vi "GeoData.vi"() -> ()   [LabVIEW 2017] (continued)
H1\n47264\t18105\tNorman\tIN\tMonroe County\tH1\n47460\t18105\tSpencer\tIN\tMonroe County\tH1\n47426\t18105\tClear creek\tIN\tMonroe County\tH1\n47434\t18105\tHarrodsburg\tIN\tMonroe County\tH1\n47463\t18105\tStanford\tIN\tMonroe County\tH1\n47458\t18105\tSmithville\tIN\tMonroe County\tH1\n47402\t18105\tBloomington\tIN\tMonroe County\tH1\n46151\t18105\tMartinsville\tIN\tMonroe County\tH1\n47990\t18107\tWaynetown\tIN\tMontgomery County\tH1\n46035\t18107\tColfax\tIN\tMontgomery County\tH1\n47954\t18107\tLadoga\tIN\tMontgomery County\tH1\n46175\t18107\tRussellville\tIN\tMontgomery County\tH1\n47955\t18107\tLinden\tIN\tMontgomery County\tH1\n47933\t18107\tCrawfordsville\tIN\tMontgomery County\tH1\n47968\t18107\tNew ross\tIN\tMontgomery County\tH1\n47967\t18107\tNew richmond\tIN\tMontgomery County\tH1\n47994\t18107\tWingate\tIN\tMontgomery County\tH1\n47949\t18107\tHillsboro\tIN\tMontgomery County\tH1\n47916\t18107\tAlamo\tIN\tMontgomery County\tH1\n47981\t18107\tRomney\tIN\tMontgomery County\tH1\n47940\t18107\tDarlington\tIN\tMontgomery County\tH1\n47989\t18107\tWaveland\tIN\tMontgomery County\tH1\n46071\t18107\tThorntown\tIN\tMontgomery County\tH1\n47930\t18107\tClarks hill\tIN\tMontgomery County\tH1\n47965\t18107\tNew market\tIN\tMontgomery County\tH1\n46158\t18109\tMooresville\tIN\tMorgan County\tH1\n46166\t18109\tParagon\tIN\tMorgan County\tH1\n46106\t18109\tBargersville\tIN\tMorgan County\tH1\n47433\t18109\tGosport\tIN\tMorgan County\tH1\n46120\t18109\tCloverdale\tIN\tMorgan County\tH1\n46111\t18109\tBrooklyn\tIN\tMorgan County\tH1\n46157\t18109\tMonrovia\tIN\tMorgan County\tH1\n46113\t18109\tCamby\tIN\tMorgan County\tH1\n46125\t18109\tEminence\tIN\tMorgan County\tH1\n46180\t18109\tStilesville\tIN\tMorgan County\tH1\n46160\t18109\tMorgantown\tIN\tMorgan County\tH1\n46118\t18109\tClayton\tIN\tMorgan County\tH1\n46151\t18109\tMartinsville\tIN\tMorgan County\tH1\n47456\t18109\tQuincy\tIN\tMorgan County\tH1\n46310\t18111\tDemotte\tIN\tNewton County\tH1\n46379\t18111\tSumava resorts\tIN\tNewton County\tH1\n46372\t18111\tRoselawn\tIN\tNewton County\tH1\n46349\t18111\tLake village\tIN\tNewton County\tH1\n47978\t18111\tRensselaer\tIN\tNewton County\tH1\n46341\t18111\tHebron\tIN\tNewton County\tH1\n47948\t18111\tGoodland\tIN\tNewton County\tH1\n47942\t18111\tEarl park\tIN\tNewton County\tH1\n47922\t18111\tBrook\tIN\tNewton County\tH1\n47963\t18111\tMorocco\tIN\tNewton County\tH1\n47964\t18111\tMount ayr\tIN\tNewton County\tH1\n46381\t18111\tThayer\tIN\tNewton County\tH1\n47951\t18111\tKentland\tIN\tNewton County\tH1\n47943\t18111\tFair oaks\tIN\tNewton County\tH1\n46725\t18113\tColumbia city\tIN\tNoble County\tH1\n46760\t18113\tKimmell\tIN\tNoble County\tH1\n46732\t18113\tCromwell\tIN\tNoble County\tH1\n46796\t18113\tWolflake\tIN\tNoble County\tH1\n46730\t18113\tCorunna\tIN\tNoble County\tH1\n46748\t18113\tHuntertown\tIN\tNoble County\tH1\n46794\t18113\tWawaka\tIN\tNoble County\tH1\n46562\t18113\tPierceton\tIN\tNoble County\tH1\n46755\t18113\tKendallville\tIN\tNoble County\tH1\n46571\t18113\tTopeka\tIN\tNoble County\tH1\n46764\t18113\tLarwill\tIN\tNoble County\tH1\n46701\t18113\tAlbion\tIN\tNoble County\tH1\n46710\t18113\tAvilla\tIN\tNoble County\tH1\n46784\t18113\tRome city\tIN\tNoble County\tH1\n46543\t18113\tMillersburg\tIN\tNoble County\tH1\n46763\t18113\tLaotto\tIN\tNoble County\tH1\n46767\t18113\tLigonier\tIN\tNoble County\tH1\n46723\t18113\tChurubusco\tIN\tNoble County\tH1\n46795\t18113\tWolcottville\tIN\tNoble County\tH1\n47001\t18115\tAurora\tIN\tOhio County\tH1\n47018\t18115\tDillsboro\tIN\tOhio County\tH1\n47038\t18115\tPatriot\tIN\tOhio County\tH1\n47011\t18115\tBennington\tIN\tOhio County\tH1\n47040\t18115\tRising sun\tIN\tOhio County\tH1\n47017\t18115\tCross plains\tIN\tOhio County\tH1\n47108\t18117\tCampbellsburg\tIN\tOrange County\tH1\n47175\t18117\tTaswell\tIN\tOrange County\tH1\n47469\t18117\tWest baden springs\tIN\tOrange County\tH1\n47452\t18117\tOrleans\tIN\tOrange County\tH1\n47446\t18117\tMitchell\tIN\tOrange County\tH1\n47454\t18117\tPaoli\tIN\tOrange County\tH1\n47125\t18117\tHardinsburg\tIN\tOrange County\tH1\n47581\t18117\tShoals\tIN\tOrange County\tH1\n47527\t18117\tDubois\tIN\tOrange County\tH1\n47140\t18117\tMarengo\tIN\tOrange County\tH1\n47118\t18117\tEnglish\tIN\tOrange County\tH1\n47432\t18117\tFrench lick\tIN\tOrange County\tH1\n47513\t18117\tBirdseye\tIN\tOrange County\tH1\n46166\t18119\tParagon\tIN\tOwen County\tH1\n47433\t18119\tGosport\tIN\tOwen County\tH1\n46120\t18119\tCloverdale\tIN\tOwen County\tH1\n47424\t18119\tBloomfield\tIN\tOwen County\tH1\n47471\t18119\tWorthington\tIN\tOwen County\tH1\n47868\t18119\tPoland\tIN\tOwen County\tH1\n47427\t18119\tCoal city\tIN\tOwen County\tH1\n47459\t18119\tSolsberry\tIN\tOwen County\tH1\n47841\t18119\tClay city\tIN\tOwen County\tH1\n47404\t18119\tBloomington\tIN\tOwen County\tH1\n47431\t18119\tFreedom\tIN\tOwen County\tH1\n47460\t18119\tSpencer\tIN\tOwen County\tH1\n47455\t18119\tPatricksburg\tIN\tOwen County\tH1\n47456\t18119\tQuincy\tIN\tOwen County\tH1\n47833\t18119\tBowling green\tIN\tOwen County\tH1\n46135\t18121\tGreencastle\tIN\tParke County\tH1\n47952\t18121\tKingman\tIN\tParke County\tH1\n47859\t18121\tMarshall\tIN\tParke County\tH1\n47832\t18121\tBloomingdale\tIN\tParke County\tH1\n46175\t18121\tRussellville\tIN\tParke County\tH1\n47834\t18121\tBrazil\tIN\tParke County\tH1\n47872\t18121\tRockville\tIN\tParke County\tH1\n47860\t18121\tMecca\tIN\tParke County\tH1\n47836\t18121\tBridgeton\tIN\tParke County\tH1\n47874\t18121\tRosedale\tIN\tParke County\tH1\n47989\t18121\tWaveland\tIN\tParke County\tH1\n47805\t18121\tTerre haute\tIN\tParke County\tH1\n47837\t18121\tCarbon\tIN\tParke County\tH1\n47862\t18121\tMontezuma\tIN\tParke County\tH1\n47588\t18123\tTroy\tIN\tPerry County\tH1\n47525\t18123\tDerby\tIN\tPerry County\tH1\n47576\t18123\tSaint croix\tIN\tPerry County\tH1\n47515\t18123\tBristow\tIN\tPerry County\tH1\n47574\t18123\tRome\tIN\tPerry County\tH1\n47586\t18123\tTell city\tIN\tPerry County\tH1\n47551\t18123\tLeopold\tIN\tPerry County\tH1\n47514\t18123\tBranchville\tIN\tPerry County\tH1\n47137\t18123\tLeavenworth\tIN\tPerry County\tH1\n47118\t18123\tEnglish\tIN\tPerry County\tH1\n47520\t18123\tCannelton\tIN\tPerry County\tH1\n47577\t18123\tSaint meinrad\tIN\tPerry County\tH1\n47532\t18123\tFerdinand\tIN\tPerry County\tH1\n47513\t18123\tBirdseye\tIN\tPerry County\tH1\n47660\t18125\tOakland city\tIN\tPike County\tH1\n47666\t18125\tPatoka\tIN\tPike County\tH1\n47598\t18125\tWinslow\tIN\tPike County\tH1\n47542\t18125\tHuntingburg\tIN\tPike County\tH1\n47567\t18125\tPetersburg\tIN\tPike County\tH1\n47564\t18125\tOtwell\tIN\tPike County\tH1\n47541\t18125\tHolland\tIN\tPike County\tH1\n47590\t18125\tVelpen\tIN\tPike County\tH1\n47619\t18125\tLynnville\tIN\tPike County\tH1\n47585\t18125\tStendal\tIN\tPike County\tH1\n47640\t18125\tHazleton\tIN\tPike County\tH1\n47584\t18125\tSpurgeon\tIN\tPike County\tH1\n46301\t18127\tBeverly shores\tIN\tPorter County\tH1\n46391\t18127\tWestville\tIN\tPorter County\tH1\n46385\t18127\tValparaiso\tIN\tPorter County\tH1\n46384\t18127\tValparaiso\tIN\tPorter County\tH1\n46347\t18127\tKouts\tIN\tPorter County\tH1\n46403\t18127\tGary\tIN\tPorter County\tH1\n46341\t18127\tHebron\tIN\tPorter County\tH1\n46307\t18127\tCrown point\tIN\tPorter County\tH1\n46304\t18127\tChesterton\tIN\tPorter County\tH1\n46383\t18127\tValparaiso\tIN\tPorter County\tH1\n46368\t18127\tPortage\tIN\tPorter County\tH1\n46348\t18127\tLa crosse\tIN\tPorter County\tH1\n46342\t18127\tHobart\tIN\tPorter County\tH1\n46360\t18127\tMichigan city\tIN\tPorter County\tH1\n46302\t18127\tBoone grove\tIN\tPorter County\tH1\n46393\t18127\tWheeler\tIN\tPorter County\tH1\n47620\t18129\tMount vernon\tIN\tPosey County\tH1\n47633\t18129\tPoseyville\tIN\tPosey County\tH1\n47616\t18129\tGriffin\tIN\tPosey County\tH1\n47638\t18129\tWadesville\tIN\tPosey County\tH1\n47712\t18129\tEvansville\tIN\tPosey County\tH1\n47631\t18129\tNew harmony\tIN\tPosey County\tH1\n47720\t18129\tEvansville\tIN\tPosey County\tH1\n47612\t18129\tCynthiana\tIN\tPosey County\tH1\n47960\t18131\tMonticello\tIN\tPulaski County\tH1\n47959\t18131\tMonon\tIN\tPulaski County\tH1\n46374\t18131\tSan pierre\tIN\tPulaski County\tH1\n46985\t18131\tStar city\tIN\tPulaski County\tH1\n46978\t18131\tRoyal center\tIN\tPulaski County\tH1\n47946\t18131\tFrancesville\tIN\tPulaski County\tH1\n46366\t18131\tNorth judson\tIN\tPulaski County\tH1\n46960\t18131\tMonterey\tIN\tPulaski County\tH1\n47957\t18131\tMedaryville\tIN\tPulaski County\tH1\n46968\t18131\tOra\tIN\tPulaski County\tH1\n46511\t18131\tCulver\tIN\tPulaski County\tH1\n46939\t18131\tKewanna\tIN\tPulaski County\tH1\n46996\t18131\tWinamac\tIN\tPulaski County\tH1\n47840\t18133\tCenterpoint\tIN\tPutnam County\tH1\n46171\t18133\tReelsville\tIN\tPutnam County\tH1\n46135\t18133\tGreencastle\tIN\tPutnam County\tH1\n46120\t18133\tCloverdale\tIN\tPutnam County\tH1\n47954\t18133\tLadoga\tIN\tPutnam County\tH1\n46175\t18133\tRussellville\tIN\tPutnam County\tH1\n47868\t18133\tPoland\tIN\tPutnam County\tH1\n46170\t18133\tPutnamville\tIN\tPutnam County\tH1\n46172\t18133\tRoachdale\tIN\tPutnam County\tH1\n47834\t18133\tBrazil\tIN\tPutnam County\tH1\n47872\t18133\tRockville\tIN\tPutnam County\tH1\n46165\t18133\tNorth salem\tIN\tPutnam County\tH1\n46128\t18133\tFillmore\tIN\tPutnam County\tH1\n47989\t18133\tWaveland\tIN\tPutnam County\tH1\n46121\t18133\tCoatesville\tIN\tPutnam County\tH1\n46105\t18133\tBainbridge\tIN\tPutnam County\tH1\n47456\t18133\tQuincy\tIN\tPutnam County\tH1\n47355\t18135\tLynn\tIN\tRandolph County\tH1\n47390\t18135\tUnion city\tIN\tRandolph County\tH1\n47393\t18135\tWilliamsburg\tIN\tRandolph County\tH1\n47373\t18135\tRedkey\tIN\tRandolph County\tH1\n47320\t18135\tAlbany\tIN\tRandolph County\tH1\n47380\t18135\tRidgeville\tIN\tRandolph County\tH1\n47358\t18135\tModoc\tIN\tRandolph County\tH1\n47383\t18135\tSelma\tIN\tRandolph County\tH1\n47394\t18135\tWinchester\tIN\tRandolph County\tH1\n47340\t18135\tFarmland\tIN\tRandolph County\tH1\n47341\t18135\tFountain city\tIN\tRandolph County\tH1\n47368\t18135\tParker city\tIN\tRandolph County\tH1\n47354\t18135\tLosantville\tIN\tRandolph County\tH1\n47382\t18135\tSaratoga\tIN\tRandolph County\tH1\n47224\t18137\tCanaan\tIN\tRipley County\tH1\n47018\t18137\tDillsboro\tIN\tRipley County\tH1\n47240\t18137\tGreensburg\tIN\tRipley County\tH1\n47039\t18137\tPierceville\tIN\tRipley County\tH1\n47042\t18137\tVersailles\tIN\tRipley County\tH1\n47032\t18137\tMoores hill\tIN\tRipley County\tH1\n47034\t18137\tNapoleon\tIN\tRipley County\tH1\n47023\t18137\tHolton\tIN\tRipley County\tH1\n47223\t18137\tButlerville\tIN\tRipley County\tH1\n47006\t18137\tBatesville\tIN\tRipley County\tH1\n47017\t18137\tCross plains\tIN\tRipley County\tH1\n47250\t18137\tMadison\tIN\tRipley County\tH1\n47033\t18137\tMorris\tIN\tRipley County\tH1\n47037\t18137\tOsgood\tIN\tRipley County\tH1\n47041\t18137\tSunman\tIN\tRipley County\tH1\n47021\t18137\tFriendship\tIN\tRipley County\tH1\n47031\t18137\tMilan\tIN\tRipley County\tH1\n46156\t18139\tMilroy\tIN\tRush County\tH1\n47240\t18139\tGreensburg\tIN\tRush County\tH1\n46148\t18139\tKnightstown\tIN\tRush County\tH1\n46115\t18139\tCarthage\tIN\tRush County\tH1\n46155\t18139\tMays\tIN\tRush County\tH1\n46127\t18139\tFalmouth\tIN\tRush County\tH1\n46176\t18139\tShelbyville\tIN\tRush County\tH1\n46150\t18139\tManilla\tIN\tRush County\tH1\n47352\t18139\tLewisville\tIN\tRush County\tH1\n46173\t18139\tRushville\tIN\tRush County\tH1\n46133\t18139\tGlenwood\tIN\tRush County\tH1\n47272\t18139\tSaint paul\tIN\tRush County\tH1\n46140\t18139\tGreenfield\tIN\tRush County\tH1\n46161\t18139\tMorristown\tIN\tRush County\tH1\n46182\t18139\tWaldron\tIN\tRush County\tH1\n46146\t18139\tHomer\tIN\tRush County\tH1\n46104\t18139\tArlington\tIN\tRush County\tH1\n46613\t18141\tSouth bend\tIN\tSt. Joseph County\tH1\n46628\t18141\tSouth bend\tIN\tSt. Joseph County\tH1\n46680\t18141\tSouth bend\tIN\tSt. Joseph County\tH1\n46595\t18141\tWyatt\tIN\tSt. Joseph County\tH1\n46536\t18141\tLakeville\tIN\tSt. Joseph County\tH1\n46561\t18141\tOsceola\tIN\tSt. Joseph County\tH1\n46552\t18141\tNew carlisle\tIN\tSt. Joseph County\tH1\n46546\t18141\tMishawaka\tIN\tSt. Joseph County\tH1\n46550\t18141\tNappanee\tIN\tSt. Joseph County\tH1\n46616\t18141\tSouth bend\tIN\tSt. Joseph County\tH1\n46660\t18141\tSouth bend\tIN\tSt. Joseph County\tH1\n46563\t18141\tPlymouth\tIN\tSt. Joseph County\tH1\n46506\t18141\tBremen\tIN\tSt. Joseph County\tH1\n46556\t18141\tNotre dame\tIN\tSt. Joseph County\tH1\n46617\t18141\tSouth bend\tIN\tSt. Joseph County\tH1\n46601\t18141\tSouth bend\tIN\tSt. Joseph County\tH1\n46626\t18141\tSouth bend\tIN\tSt. Joseph County\tH1\n46554\t18141\tNorth liberty\tIN\tSt. Joseph County\tH1\n46517\t18141\tElkhart\tIN\tSt. Joseph County\tH1\n46530\t18141\tGranger\tIN\tSt. Joseph County\tH1\n46614\t18141\tSouth bend\tIN\tSt. Joseph County\tH1\n46615\t18141\tSouth bend\tIN\tSt. Joseph County\tH1\n46624\t18141\tSouth bend\tIN\tSt. Joseph County\tH1\n46544\t18141\tMishawaka\tIN\tSt. Joseph County\tH1\n46545\t18141\tMishawaka\tIN\tSt. Joseph County\tH1\n46619\t18141\tSouth bend\tIN\tSt. Joseph County\tH1\n46637\t18141\tSouth bend\tIN\tSt. Joseph County\tH1\n46573\t18141\tWakarusa\tIN\tSt. Joseph County\tH1\n46574\t18141\tWalkerton\tIN\tSt. Joseph County\tH1\n46634\t18141\tSouth bend\tIN\tSt. Joseph County\tH1\n46635\t18141\tSouth bend\tIN\tSt. Joseph County\tH1\n47141\t18143\tMarysville\tIN\tScott County\tH1\n47102\t18143\tAustin\tIN\tScott County\tH1\n47147\t18143\tNabb\tIN\tScott County\tH1\n47170\t18143\tScottsburg\tIN\tScott County\tH1\n47126\t18143\tHenryville\tIN\tScott County\tH1\n47138\t18143\tLexington\tIN\tScott County\tH1\n47177\t18143\tUnderwood\tIN\tScott County\tH1\n47230\t18143\tDeputy\tIN\tScott County\tH1\n47240\t18145\tGreensburg\tIN\tShelby County\tH1\n46144\t18145\tGwynneville\tIN\tShelby County\tH1\n46162\t18145\tNeedham\tIN\tShelby County\tH1\n46176\t18145\tShelbyville\tIN\tShelby County\tH1\n46130\t18145\tFountaintown\tIN\tShelby County\tH1\n46163\t18145\tNew palestine\tIN\tShelby County\tH1\n46150\t18145\tManilla\tIN\tShelby County\tH1\n46110\t18145\tBoggstown\tIN\tShelby County\tH1\n47272\t18145\tSaint paul\tIN\tShelby County\tH1\n46140\t18145\tGreenfield\tIN\tShelby County\tH1\n46161\t18145\tMorristown\tIN\tShelby County\tH1\n46182\t18145\tWaldron\tIN\tShelby County\tH1\n46131\t18145\tFranklin\tIN\tShelby County\tH1\n46124\t18145\tEdinburgh\tIN\tShelby County\tH1\n46126\t18145\tFairland\tIN\tShelby County\tH1\n46259\t18145\tIndianapolis\tIN\tShelby County\tH1\n47234\t18145\tFlat rock\tIN\tShelby County\tH1\n47523\t18147\tDale\tIN\tSpencer County\tH1\n47588\t18147\tTroy\tIN\tSpencer County\tH1\n47617\t18147\tHatfield\tIN\tSpencer County\tH1\n47531\t18147\tEvanston\tIN\tSpencer County\tH1\n47611\t18147\tChrisney\tIN\tSpencer County\tH1\n47550\t18147\tLamar\tIN\tSpencer County\tH1\n47536\t18147\tFulda\tIN\tSpencer County\tH1\n47556\t18147\tMariah hill\tIN\tSpencer County\tH1\n47615\t18147\tGrandview\tIN\tSpencer County\tH1\n47579\t18147\tSanta claus\tIN\tSpencer County\tH1\n47635\t18147\tRockport\tIN\tSpencer County\tH1\n47637\t18147\tTennyson\tIN\tSpencer County\tH1\n47634\t18147\tRichland\tIN\tSpencer County\tH1\n47541\t18147\tHolland\tIN\tSpencer County\tH1\n47552\t18147\tLincoln city\tIN\tSpencer County\tH1\n47601\t18147\tBoonville\tIN\tSpencer County\tH1\n47537\t18147\tGentryville\tIN\tSpencer County\tH1\n47577\t18147\tSaint meinrad\tIN\tSpencer County\tH1\n47532\t18147\tFerdinand\tIN\tSpencer County\tH1\n46374\t18149\tSan pierre\tIN\tStarke County\tH1\n46563\t18149\tPlymouth\tIN\tStarke County\tH1\n46366\t18149\tNorth judson\tIN\tStarke County\tH1\n46534\t18149\tKnox\tIN\tStarke County\tH1\n46531\t18149\tGrovertown\tIN\tStarke County\tH1\n46960\t18149\tMonterey\tIN\tStarke County\tH1\n46968\t18149\tOra\tIN\tStarke County\tH1\n46532\t18149\tHamlet\tIN\tStarke County\tH1\n46574\t18149\tWalkerton\tIN\tStarke County\tH1\n46511\t18149\tCulver\tIN\tStarke County\tH1\n46996\t18149\tWinamac\tIN\tStarke County\tH1\n46737\t18151\tFremont\tIN\tSteuben County\tH1\n46703\t18151\tAngola\tIN\tSteuben County\tH1\n46747\t18151\tHudson\tIN\tSteuben County\tH1\n46742\t18151\tHamilton\tIN\tSteuben County\tH1\n46730\t18151\tCorunna\tIN\tSteuben County\tH1\n46776\t18151\tOrland\tIN\tSteuben County\tH1\n46793\t18151\tWaterloo\tIN\tSteuben County\tH1\n46761\t18151\tLagrange\tIN\tSteuben County\tH1\n46705\t18151\tAshley\tIN\tSteuben County\tH1\n46779\t18151\tPleasant lake\tIN\tSteuben County\tH1\n46795\t18151\tWolcottville\tIN\tSteuben County\tH1\n47850\t18153\tFarmersburg\tIN\tSullivan County\tH1\n47855\t18153\tHymera\tIN\tSullivan County\tH1\n47852\t18153\tGraysville\tIN\tSullivan County\tH1\n47528\t18153\tEdwardsport\tIN\tSullivan County\tH1\n47858\t18153\tLewis\tIN\tSullivan County\tH1\n47848\t18153\tDugger\tIN\tSullivan County\tH1\n47849\t18153\tFairbanks\tIN\tSullivan County\tH1\n47879\t18153\tShelburn\tIN\tSullivan County\tH1\n47882\t18153\tSullivan\tIN\tSullivan County\tH1\n47561\t18153\tOaktown\tIN\tSullivan County\tH1\n47438\t18153\tJasonville\tIN\tSullivan County\tH1\n47838\t18153\tCarlisle\tIN\tSullivan County\tH1\n47578\t18153\tSandborn\tIN\tSullivan County\tH1\n47861\t18153\tMerom\tIN\tSullivan County\tH1\n47866\t18153\tPimento\tIN\tSullivan County\tH1\n47224\t18155\tCanaan\tIN\tSwitzerland County\tH1\n47018\t18155\tDillsboro\tIN\tSwitzerland County\tH1\n47038\t18155\tPatriot\tIN\tSwitzerland County\tH1\n47043\t18155\tVevay\tIN\tSwitzerland County\tH1\n47011\t18155\tBennington\tIN\tSwitzerland County\tH1\n47040\t18155\tRising sun\tIN\tSwitzerland County\tH1\n47019\t18155\tEast enterprise\tIN\tSwitzerland County\tH1\n47017\t18155\tCross plains\tIN\tSwitzerland County\tH1\n47250\t18155\tMadison\tIN\tSwitzerland County\tH1\n47020\t18155\tFlorence\tIN\tSwitzerland County\tH1\n47901\t18157\tLafayette\tIN\tTippecanoe County\tH1\n47902\t18157\tLafayette\tIN\tTippecanoe County\tH1\n47903\t18157\tLafayette\tIN\tTippecanoe County\tH1\n47924\t18157\tBuck creek\tIN\tTippecanoe County\tH1\n47941\t18157\tDayton\tIN\tTippecanoe County\tH1\n46041\t18157\tFrankfort\tIN\tTippecanoe County\tH1\n47992\t18157\tWestpoint\tIN\tTippecanoe County\tH1\n47907\t18157\tWest lafayette\tIN\tTippecanoe County\tH1\n47962\t18157\tMontmorenci\tIN\tTippecanoe County\tH1\n47955\t18157\tLinden\tIN\tTippecanoe County\tH1\n47970\t18157\tOtterbein\tIN\tTippecanoe County\tH1\n47996\t18157\tWest lafayette\tIN\tTippecanoe County\tH1\n47905\t18157\tLafayette\tIN\tTippecanoe County\tH1\n47906\t18157\tWest lafayette\tIN\tTippecanoe County\tH1\n47909\t18157\tLafayette\tIN\tTippecanoe County\tH1\n47904\t18157\tLafayette\tIN\tTippecanoe County\tH1\n47967\t18157\tNew richmond\tIN\tTippecanoe County\tH1\n47994\t18157\tWingate\tIN\tTippecanoe County\tH1\n47983\t18157\tStockwell\tIN\tTippecanoe County\tH1\n47920\t18157\tBattle ground\tIN\tTippecanoe County\tH1\n46058\t18157\tMulberry\tIN\tTippecanoe County\tH1\n47981\t18157\tRomney\tIN\tTippecanoe County\tH1\n46923\t18157\tDelphi\tIN\tTippecanoe County\tH1\n47930\t18157\tClarks hill\tIN\tTippecanoe County\tH1\n47918\t18157\tAttica\tIN\tTippecanoe County\tH1\n46902\t18159\tKokomo\tIN\tTipton County\tH1\n46031\t18159\tAtlanta\tIN\tTipton County\tH1\n46076\t18159\tWindfall\tIN\tTipton County\tH1\n46069\t18159\tSheridan\tIN\tTipton County\tH1\n46045\t18159\tGoldsmith\tIN\tTipton County\tH1\n46068\t18159\tSharpsville\tIN\tTipton County\tH1\n46047\t18159\tHobbs\tIN\tTipton County\tH1\n46036\t18159\tElwood\tIN\tTipton County\tH1\n46049\t18159\tKempton\tIN\tTipton County\tH1\n46072\t18159\tTipton\tIN\tTipton County\tH1\n46050\t18159\tKirklin\tIN\tTipton County\tH1\n46979\t18159\tRussiaville\tIN\tTipton County\tH1\n47331\t18161\tConnersville\tIN\tUnion County\tH1\n47010\t18161\tBath\tIN\tUnion County\tH1\n47353\t18161\tLiberty\tIN\tUnion County\tH1\n47003\t18161\tWest college corner\tIN\tUnion County\tH1\n47325\t18161\tBrownsville\tIN\tUnion County\tH1\n47633\t18163\tPoseyville\tIN\tVanderburgh County\tH1\n47706\t18163\tEvansville\tIN\tVanderburgh County\tH1\n47708\t18163\tEvansville\tIN\tVanderburgh County\tH1\n47702\t18163\tEvansville\tIN\tVanderburgh County\tH1\n47705\t18163\tEvansville\tIN\tVanderburgh County\tH1\n47721\t18163\tEvansville\tIN\tVanderburgh County\tH1\n47736\t18163\tEvansville\tIN\tVanderburgh County\tH1\n47722\t18163\tEvansville\tIN\tVanderburgh County\tH1\n47747\t18163\tEvansville\tIN\tVanderburgh County\tH1\n47613\t18163\tElberfeld\tIN\tVanderburgh County\tH1\n47711\t18163\tEvansville\tIN\tVanderburgh County\tH1\n47638\t18163\tWadesville\tIN\tVanderburgh County\tH1\n47712\t18163\tEvansville\tIN\tVanderburgh County\tH1\n47735\t18163\tEvansville\tIN\tVanderburgh County\tH1\n47725\t18163\tEvansville\tIN\tVanderburgh County\tH1\n47716\t18163\tEvansville\tIN\tVanderburgh County\tH1\n47720\t18163\tEvansville\tIN\tVanderburgh County\tH1\n47710\t18163\tEvansville\tIN\tVanderburgh County\tH1\n47731\t18163\tEvansville\tIN\tVanderburgh County\tH1\n47730\t18163\tEvansville\tIN\tVanderburgh County\tH1\n47750\t18163\tEvansville\tIN\tVanderburgh County\tH1\n47714\t18163\tEvansville\tIN\tVanderburgh County\tH1\n47728\t18163\tEvansville\tIN\tVanderburgh County\tH1\n47612\t18163\tCynthiana\tIN\tVanderburgh County\tH1\n47704\t18163\tEvansville\tIN\tVanderburgh County\tH1\n47618\t18163\tInglefield\tIN\tVanderburgh County\tH1\n47639\t18163\tHaubstadt\tIN\tVanderburgh County\tH1\n47701\t18163\tEvansville\tIN\tVanderburgh County\tH1\n47734\t18163\tEvansville\tIN\tVanderburgh County\tH1\n47719\t18163\tEvansville\tIN\tVanderburgh County\tH1\n47724\t18163\tEvansville\tIN\tVanderburgh County\tH1\n47732\t18163\tEvansville\tIN\tVanderburgh County\tH1\n47737\t18163\tEvansville\tIN\tVanderburgh County\tH1\n47715\t18163\tEvansville\tIN\tVanderburgh County\tH1\n47713\t18163\tEvansville\tIN\tVanderburgh County\tH1\n47733\t18163\tEvansville\tIN\tVanderburgh County\tH1\n47703\t18163\tEvansville\tIN\tVanderburgh County\tH1\n47854\t18165\tHillsdale\tIN\tVermillion County\tH1\n47875\t18165\tSaint bernice\tIN\tVermillion County\tH1\n47831\t18165\tBlanford\tIN\tVermillion County\tH1\n47932\t18165\tCovington\tIN\tVermillion County\tH1\n47885\t18165\tWest terre haute\tIN\tVermillion County\tH1\n47966\t18165\tNewport\tIN\tVermillion County\tH1\n47884\t18165\tUniversal\tIN\tVermillion County\tH1\n47928\t18165\tCayuga\tIN\tVermillion County\tH1\n47974\t18165\tPerrysville\tIN\tVermillion County\tH1\n47842\t18165\tClinton\tIN\tVermillion County\tH1\n47847\t18165\tDana\tIN\tVermillion County\tH1\n47802\t18167\tTerre haute\tIN\tVigo County\tH1\n47863\t18167\tNew goshen\tIN\tVigo County\tH1\n47850\t18167\tFarmersburg\tIN\tVigo County\tH1\n47869\t18167\tPrairie creek\tIN\tVigo County\tH1\n47809\t18167\tTerre haute\tIN\tVigo County\tH1\n47885\t18167\tWest terre haute\tIN\tVigo County\tH1\n47858\t18167\tLewis\tIN\tVigo County\tH1\n47878\t18167\tSeelyville\tIN\tVigo County\tH1\n47834\t18167\tBrazil\tIN\tVigo County\tH1\n47803\t18167\tTerre haute\tIN\tVigo County\tH1\n47870\t18167\tPrairieton\tIN\tVigo County\tH1\n47880\t18167\tShepardsville\tIN\tVigo County\tH1\n47807\t18167\tTerre haute\tIN\tVigo County\tH1\n47804\t18167\tTerre haute\tIN\tVigo County\tH1\n47876\t18167\tSaint mary of the woods\tIN\tVigo County\tH1\n47874\t18167\tRosedale\tIN\tVigo County\tH1\n47846\t18167\tCory\tIN\tVigo County\tH1\n47871\t18167\tRiley\tIN\tVigo County\tH1\n47842\t18167\tClinton\tIN\tVigo County\tH1\n47801\t18167\tTerre haute\tIN\tVigo County\tH1\n47805\t18167\tTerre haute\tIN\tVigo County\tH1\n47866\t18167\tPimento\tIN\tVigo County\tH1\n47851\t18167\tFontanet\tIN\tVigo County\tH1\n46919\t18169\tConverse\tIN\tWabash County\tH1\n46980\t18169\tServia\tIN\tWabash County\tH1\n46974\t18169\tRoann\tIN\tWabash County\tH1\n46946\t18169\tLiberty mills\tIN\tWabash County\tH1\n46750\t18169\tHuntington\tIN\tWabash County\tH1\n46926\t18169\tDenver\tIN\tWabash County\tH1\n46941\t18169\tLagro\tIN\tWabash County\tH1\n46984\t18169\tSomerset\tIN\tWabash County\tH1\n46952\t18169\tMarion\tIN\tWabash County\tH1\n46982\t18169\tSilver lake\tIN\tWabash County\tH1\n46962\t18169\tNorth manchester\tIN\tWabash County\tH1\n46990\t18169\tUrbana\tIN\tWabash County\tH1\n46787\t18169\tSouth whitley\tIN\tWabash County\tH1\n46992\t18169\tWabash\tIN\tWabash County\tH1\n46940\t18169\tLa fontaine\tIN\tWabash County\tH1\n46702\t18169\tAndrews\tIN\tWabash County\tH1\n46970\t18169\tPeru\tIN\tWabash County\tH1\n46943\t18169\tLaketon\tIN\tWabash County\tH1\n46911\t18169\tAmboy\tIN\tWabash County\tH1\n47991\t18171\tWest lebanon\tIN\tWarren County\tH1\n47944\t18171\tFowler\tIN\tWarren County\tH1\n47917\t18171\tAmbia\tIN\tWarren County\tH1\n47993\t18171\tWilliamsport\tIN\tWarren County\tH1\n47975\t18171\tPine village\tIN\tWarren County\tH1\n47932\t18171\tCovington\tIN\tWarren County\tH1\n47970\t18171\tOtterbein\tIN\tWarren County\tH1\n47906\t18171\tWest lafayette\tIN\tWarren County\tH1\n47921\t18171\tBoswell\tIN\tWarren County\tH1\n47982\t18171\tState line\tIN\tWarren County\tH1\n47918\t18171\tAttica\tIN\tWarren County\tH1\n47660\t18173\tOakland city\tIN\tWarrick County\tH1\n47523\t18173\tDale\tIN\tWarrick County\tH1\n47613\t18173\tElberfeld\tIN\tWarrick County\tH1\n47629\t18173\tNewburgh\tIN\tWarrick County\tH1\n47610\t18173\tChandler\tIN\tWarrick County\tH1\n47630\t18173\tNewburgh\tIN\tWarrick County\tH1\n47637\t18173\tTennyson\tIN\tWarrick County\tH1\n47639\t18173\tHaubstadt\tIN\tWarrick County\tH1\n47541\t18173\tHolland\tIN\tWarrick County\tH1\n47601\t18173\tBoonville\tIN\tWarrick County\tH1\n47619\t18173\tLynnville\tIN\tWarrick County\tH1\n47537\t18173\tGentryville\tIN\tWarrick County\tH1\n47108\t18175\tCampbellsburg\tIN\tWashington County\tH1\n47167\t18175\tSalem\tIN\tWashington County\tH1\n47164\t18175\tPalmyra\tIN\tWashington County\tH1\n47281\t18175\tVallonia\tIN\tWashington County\tH1\n47452\t18175\tOrleans\tIN\tWashington County\tH1\n47165\t18175\tPekin\tIN\tWashington County\tH1\n47170\t18175\tScottsburg\tIN\tWashington County\tH1\n47125\t18175\tHardinsburg\tIN\tWashington County\tH1\n47145\t18175\tMilltown\tIN\tWashington County\tH1\n47115\t18175\tDepauw\tIN\tWashington County\tH1\n47126\t18175\tHenryville\tIN\tWashington County\tH1\n47106\t18175\tBorden\tIN\tWashington County\tH1\n47120\t18175\tFredericksburg\tIN\tWashington County\tH1\n47346\t18177\tHagerstown\tIN\tWayne County\tH1\n47331\t18177\tConnersville\tIN\tWayne County\tH1\n47355\t18177\tLynn\tIN\tWayne County\tH1\n47393\t18177\tWilliamsburg\tIN\tWayne County\tH1\n47370\t18177\tPershing\tIN\tWayne County\tH1\n47375\t18177\tRichmond\tIN\tWayne County\tH1\n47345\t18177\tGreens fork\tIN\tWayne County\tH1\n47374\t18177\tRichmond\tIN\tWayne County\tH1\n47327\t18177\tCambridge city\tIN\tWayne County\tH1\n47392\t18177\tWebster\tIN\tWayne County\tH1\n47330\t18177\tCenterville\tIN\tWayne County\tH1\n47358\t18177\tModoc\tIN\tWayne County\tH1\n47324\t18177\tBoston\tIN\tWayne County\tH1\n47341\t18177\tFountain city\tIN\tWayne County\tH1\n47339\t18177\tEconomy\tIN\tWayne County\tH1\n47325\t18177\tBrownsville\tIN\tWayne County\tH1\n47357\t18177\tMilton\tIN\tWayne County\tH1\n47360\t18177\tMooreland\tIN\tWayne County\tH1\n47354\t18177\tLosantville\tIN\tWayne County\tH1\n47335\t18177\tDublin\tIN\tWayne County\tH1\n46798\t18179\tYoder\tIN\tWells County\tH1\n46819\t18179\tFort wayne\tIN\tWells County\tH1\n47359\t18179\tMontpelier\tIN\tWells County\tH1\n46991\t18179\tVan buren\tIN\tWells County\tH1\n46714\t18179\tBluffton\tIN\tWells County\tH1\n46777\t18179\tOssian\tIN\tWells County\tH1\n46783\t18179\tRoanoke\tIN\tWells County\tH1\n47326\t18179\tBryant\tIN\tWells County\tH1\n47348\t18179\tHartford city\tIN\tWells County\tH1\n46770\t18179\tMarkle\tIN\tWells County\tH1\n46778\t18179\tPetroleum\tIN\tWells County\tH1\n46740\t18179\tGeneva\tIN\tWells County\tH1\n46759\t18179\tKeystone\tIN\tWells County\tH1\n46799\t18179\tZanesville\tIN\tWells County\tH1\n46766\t18179\tLiberty center\tIN\tWells County\tH1\n46792\t18179\tWarren\tIN\tWells County\tH1\n46952\t18179\tMarion\tIN\tWells County\tH1\n46791\t18179\tUniondale\tIN\tWells County\tH1\n46731\t18179\tCraigville\tIN\tWells County\tH1\n46733\t18179\tDecatur\tIN\tWells County\tH1\n46781\t18179\tPoneto\tIN\tWells County\tH1\n47950\t18181\tIdaville\tIN\tWhite County\tH1\n47925\t18181\tBuffalo\tIN\tWhite County\tH1\n47960\t18181\tMonticello\tIN\tWhite County\tH1\n47944\t18181\tFowler\tIN\tWhite County\tH1\n47978\t18181\tRensselaer\tIN\tWhite County\tH1\n47980\t18181\tReynolds\tIN\tWhite County\tH1\n47926\t18181\tBurnettsville\tIN\tWhite County\tH1\n47959\t18181\tMonon\tIN\tWhite County\tH1\n46985\t18181\tStar city\tIN\tWhite County\tH1\n47970\t18181\tOtterbein\tIN\tWhite County\tH1\n46978\t18181\tRoyal center\tIN\tWhite County\tH1\n47946\t18181\tFrancesville\tIN\tWhite County\tH1\n47906\t18181\tWest lafayette\tIN\tWhite County\tH1\n47923\t18181\tBrookston\tIN\tWhite County\tH1\n47929\t18181\tChalmers\tIN\tWhite County\tH1\n47920\t18181\tBattle ground\tIN\tWhite County\tH1\n47977\t18181\tRemington\tIN\tWhite County\tH1\n46996\t18181\tWinamac\tIN\tWhite County\tH1\n47995\t18181\tWolcott\tIN\tWhite County\tH1\n46725\t18183\tColumbia city\tIN\tWhitley County\tH1\n46783\t18183\tRoanoke\tIN\tWhitley County\tH1\n46750\t18183\tHuntington\tIN\tWhitley County\tH1\n46562\t18183\tPierceton\tIN\tWhitley County\tH1\n46814\t18183\tFort wayne\tIN\tWhitley County\tH1\n46962\t18183\tNorth manchester\tIN\tWhitley County\tH1\n46764\t18183\tLarwill\tIN\tWhitley County\tH1\n46701\t18183\tAlbion\tIN\tWhitley County\tH1\n46787\t18183\tSouth whitley\tIN\tWhitley County\tH1\n46723\t18183\tChurubusco\tIN\tWhitley County\tH1\n46818\t18183\tFort wayne\tIN\tWhitley County\tH1\n50002\t19001\tAdair\tIA\tAdair County\tH1\n50155\t19001\tMacksburg\tIA\tAdair County\tH1\n50273\t19001\tWinterset\tIA\tAdair County\tH1\n50846\t19001\tFontanelle\tIA\tAdair County\tH1\n50858\t19001\tOrient\tIA\tAdair County\tH1\n50048\t19001\tCasey\tIA\tAdair County\tH1\n50250\t19001\tStuart\tIA\tAdair County\tH1\n50070\t19001\tDexter\tIA\tAdair County\tH1\n50020\t19001\tAnita\tIA\tAdair County\tH1\n50801\t19001\tCreston\tIA\tAdair County\tH1\n50859\t19001\tPrescott\tIA\tAdair County\tH1\n50164\t19001\tMenlo\tIA\tAdair County\tH1\n50849\t19001\tGreenfield\tIA\tAdair County\tH1\n50837\t19001\tBridgewater\tIA\tAdair County\tH1\n50857\t19003\tNodaway\tIA\tAdams County\tH1\n50839\t19003\tCarbon\tIA\tAdams County\tH1\n50853\t19003\tMassena\tIA\tAdams County\tH1\n50843\t19003\tCumberland\tIA\tAdams County\tH1\n50801\t19003\tCreston\tIA\tAdams County\tH1\n50841\t19003\tCorning\tIA\tAdams County\tH1\n50864\t19003\tVillisca\tIA\tAdams County\tH1\n50859\t19003\tPrescott\tIA\tAdams County\tH1\n50851\t19003\tLenox\tIA\tAdams County\tH1\n50837\t19003\tBridgewater\tIA\tAdams County\tH1\n52170\t19005\tWaterville\tIA\tAllamakee County\tH1\n52172\t19005\tWaukon\tIA\tAllamakee County\tH1\n52160\t19005\tNew albin\tIA\tAllamakee County\tH1\n52101\t19005\tDecorah\tIA\tAllamakee County\tH1\n52151\t19005\tLansing\tIA\tAllamakee County\tH1\n52162\t19005\tPostville\tIA\tAllamakee County\tH1\n52146\t19005\tHarpers ferry\tIA\tAllamakee County\tH1\n52159\t19005\tMonona\tIA\tAllamakee County\tH1\n52157\t19005\tMc gregor\tIA\tAllamakee County\tH1\n52156\t19005\tLuana\tIA\tAllamakee County\tH1\n52140\t19005\tDorchester\tIA\tAllamakee County\tH1\n52574\t19007\tMystic\tIA\tAppanoose County\tH1\n52593\t19007\tUdell\tIA\tAppanoose County\tH1\n52581\t19007\tPlano\tIA\tAppanoose County\tH1\n52544\t19007\tCenterville\tIA\tAppanoose County\tH1\n52555\t19007\tExline\tIA\tAppanoose County\tH1\n52549\t19007\tCincinnati\tIA\tAppanoose County\tH1\n52571\t19007\tMoravia\tIA\tAppanoose County\tH1\n52572\t19007\tMoulton\tIA\tAppanoose County\tH1\n52590\t19007\tSeymour\tIA\tAppanoose County\tH1\n52569\t19007\tMelrose\tIA\tAppanoose County\tH1\n52594\t19007\tUnionville\tIA\tAppanoose County\tH1\n50117\t19009\tHamlin\tIA\tAudubon County\tH1\n50110\t19009\tGray\tIA\tAudubon County\tH1\n50076\t19009\tExira\tIA\tAudubon County\tH1\n51440\t19009\tDedham\tIA\tAudubon County\tH1\n51531\t19009\tElk horn\tIA\tAudubon County\tH1\n51455\t19009\tManning\tIA\tAudubon County\tH1\n50020\t19009\tAnita\tIA\tAudubon County\tH1\n50042\t19009\tBrayton\tIA\tAudubon County\tH1\n50022\t19009\tAtlantic\tIA\tAudubon County\tH1\n50025\t19009\tAudubon\tIA\tAudubon County\tH1\n51543\t19009\tKimballton\tIA\tAudubon County\tH1\n51463\t19009\tTempleton\tIA\tAudubon County\tH1\n50058\t19009\tCoon rapids\tIA\tAudubon County\tH1\n50651\t19011\tLa porte city\tIA\tBenton County\tH1\n52210\t19011\tBrandon\tIA\tBenton County\tH1\n52213\t19011\tCenter point\tIA\tBenton County\tH1\n52345\t19011\tUrbana\tIA\tBenton County\tH1\n52346\t19011\tVan horne\tIA\tBenton County\tH1\n52332\t19011\tShellsburg\tIA\tBenton County\tH1\n52225\t19011\tElberon\tIA\tBenton County\tH1\n52206\t19011\tAtkins\tIA\tBenton County\tH1\n52229\t19011\tGarrison\tIA\tBenton County\tH1\n52301\t19011\tMarengo\tIA\tBenton County\tH1\n52257\t19011\tLuzerne\tIA\tBenton County\tH1\n52315\t19011\tNewhall\tIA\tBenton County\tH1\n52352\t19011\tWalker\tIA\tBenton County\tH1\n52313\t19011\tMount auburn\tIA\tBenton County\tH1\n52209\t19011\tBlairstown\tIA\tBenton County\tH1\n52404\t19011\tCedar rapids\tIA\tBenton County\tH1\n52351\t19011\tWalford\tIA\tBenton County\tH1\n52318\t19011\tNorway\tIA\tBenton County\tH1\n52224\t19011\tDysart\tIA\tBenton County\tH1\n52349\t19011\tVinton\tIA\tBenton County\tH1\n52324\t19011\tPalo\tIA\tBenton County\tH1\n52249\t19011\tKeystone\tIA\tBenton County\tH1\n52228\t19011\tFairfax\tIA\tBenton County\tH1\n52208\t19011\tBelle plaine\tIA\tBenton County\tH1\n52354\t19011\tWatkins\tIA\tBenton County\tH1\n50701\t19013\tWaterloo\tIA\tBlack Hawk County\tH1\n50707\t19013\tEvansdale\tIA\tBlack Hawk County\tH1\n50651\t19013\tLa porte city\tIA\tBlack Hawk County\tH1\n50622\t19013\tDenver\tIA\tBlack Hawk County\tH1\n50668\t19013\tReadlyn\tIA\tBlack Hawk County\tH1\n50623\t19013\tDewar\tIA\tBlack Hawk County\tH1\n50702\t19013\tWaterloo\tIA\tBlack Hawk County\tH1\n50703\t19013\tWaterloo\tIA\tBlack Hawk County\tH1\n50647\t19013\tJanesville\tIA\tBlack Hawk County\tH1\n50648\t19013\tJesup\tIA\tBlack Hawk County\tH1\n50613\t19013\tCedar falls\tIA\tBlack Hawk County\tH1\n50667\t19013\tRaymond\tIA\tBlack Hawk County\tH1\n50634\t19013\tGilbertville\tIA\tBlack Hawk County\tH1\n50669\t19013\tReinbeck\tIA\tBlack Hawk County\tH1\n50614\t19013\tCedar falls\tIA\tBlack Hawk County\tH1\n50626\t19013\tDunkerton\tIA\tBlack Hawk County\tH1\n50704\t19013\tWaterloo\tIA\tBlack Hawk County\tH1\n50629\t19013\tFairbank\tIA\tBlack Hawk County\tH1\n50675\t19013\tTraer\tIA\tBlack Hawk County\tH1\n50612\t19013\tBuckingham\tIA\tBlack Hawk County\tH1\n50643\t19013\tHudson\tIA\tBlack Hawk County\tH1\n50220\t19015\tPerry\tIA\tBoone County\tH1\n50530\t19015\tDayton\tIA\tBoone County\tH1\n50014\t19015\tAmes\tIA\tBoone County\tH1\n50212\t19015\tOgden\tIA\tBoone County\tH1\n50064\t19015\tDana\tIA\tBoone County\tH1\n50244\t19015\tSlater\tIA\tBoone County\tH1\n50235\t19015\tRippey\tIA\tBoone County\tH1\n50134\t19015\tKelley\tIA\tBoone County\tH1\n50223\t19015\tPilot mound\tIA\tBoone County\tH1\n50039\t19015\tBouton\tIA\tBoone County\tH1\n50152\t19015\tLuther\tIA\tBoone County\tH1\n50036\t19015\tBoone\tIA\tBoone County\tH1\n50249\t19015\tStratford\tIA\tBoone County\tH1\n50156\t19015\tMadrid\tIA\tBoone County\tH1\n50276\t19015\tWoodward\tIA\tBoone County\tH1\n50040\t19015\tBoxholm\tIA\tBoone County\tH1\n50248\t19015\tStory city\tIA\tBoone County\tH1\n50217\t19015\tPaton\tIA\tBoone County\tH1\n50107\t19015\tGrand junction\tIA\tBoone County\tH1\n50243\t19015\tSheldahl\tIA\tBoone County\tH1\n50031\t19015\tBeaver\tIA\tBoone County\tH1\n50622\t19017\tDenver\tIA\tBremer County\tH1\n50668\t19017\tReadlyn\tIA\tBremer County\tH1\n50677\t19017\tWaverly\tIA\tBremer County\tH1\n50647\t19017\tJanesville\tIA\tBremer County\tH1\n50613\t19017\tCedar falls\tIA\tBremer County\tH1\n50676\t19017\tTripoli\tIA\tBremer County\tH1\n50645\t19017\tIonia\tIA\tBremer County\tH1\n50670\t19017\tShell rock\tIA\tBremer County\tH1\n50674\t19017\tSumner\tIA\tBremer County\tH1\n50630\t19017\tFredericksburg\tIA\tBremer County\tH1\n50666\t19017\tPlainfield\tIA\tBremer County\tH1\n50664\t19017\tOran\tIA\tBremer County\tH1\n50631\t19017\tFrederika\tIA\tBremer County\tH1\n50629\t19017\tFairbank\tIA\tBremer County\tH1\n50658\t19017\tNashua\tIA\tBremer County\tH1\n50651\t19019\tLa porte city\tIA\tBuchanan County\tH1\n52210\t19019\tBrandon\tIA\tBuchanan County\tH1\n50662\t19019\tOelwein\tIA\tBuchanan County\tH1\n50648\t19019\tJesup\tIA\tBuchanan County\tH1\n52352\t19019\tWalker\tIA\tBuchanan County\tH1\n52330\t19019\tRyan\tIA\tBuchanan County\tH1\n50650\t19019\tLamont\tIA\tBuchanan County\tH1\n52326\t19019\tQuasqueton\tIA\tBuchanan County\tH1\n50682\t19019\tWinthrop\tIA\tBuchanan County\tH1\n50644\t19019\tIndependence\tIA\tBuchanan County\tH1\n50629\t19019\tFairbank\tIA\tBuchanan County\tH1\n52329\t19019\tRowley\tIA\tBuchanan County\tH1\n50641\t19019\tHazleton\tIA\tBuchanan County\tH1\n50607\t19019\tAurora\tIA\tBuchanan County\tH1\n50654\t19019\tMasonville\tIA\tBuchanan County\tH1\n50671\t19019\tStanley\tIA\tBuchanan County\tH1\n52218\t19019\tCoggon\tIA\tBuchanan County\tH1\n50568\t19021\tNewell\tIA\tBuena Vista County\tH1\n51047\t19021\tPeterson\tIA\tBuena Vista County\tH1\n50567\t19021\tNemaha\tIA\tBuena Vista County\tH1\n50554\t19021\tLaurens\tIA\tBuena Vista County\tH1\n51020\t19021\tGalva\tIA\tBuena Vista County\tH1\n50576\t19021\tRembrandt\tIA\tBuena Vista County\tH1\n50540\t19021\tFonda\tIA\tBuena Vista County\tH1\n51005\t19021\tAurelia\tIA\tBuena Vista County\tH1\n50565\t19021\tMarathon\tIA\tBuena Vista County\tH1\n51002\t19021\tAlta\tIA\tBuena Vista County\tH1\n51053\t19021\tSchaller\tIA\tBuena Vista County\tH1\n50510\t19021\tAlbert city\tIA\tBuena Vista County\tH1\n51366\t19021\tWebb\tIA\tBuena Vista County\tH1\n50588\t19021\tStorm lake\tIA\tBuena Vista County\tH1\n50592\t19021\tTruesdale\tIA\tBuena Vista County\tH1\n50585\t19021\tSioux rapids\tIA\tBuena Vista County\tH1\n51033\t19021\tLinn grove\tIA\tBuena Vista County\tH1\n50433\t19023\tDougherty\tIA\tButler County\tH1\n50677\t19023\tWaverly\tIA\tButler County\tH1\n50636\t19023\tGreene\tIA\tButler County\tH1\n50625\t19023\tDumont\tIA\tButler County\tH1\n50613\t19023\tCedar falls\tIA\tButler County\tH1\n50602\t19023\tAllison\tIA\tButler County\tH1\n50605\t19023\tAredale\tIA\tButler County\tH1\n50619\t19023\tClarksville\tIA\tButler County\tH1\n50670\t19023\tShell rock\tIA\tButler County\tH1\n50601\t19023\tAckley\tIA\tButler County\tH1\n50666\t19023\tPlainfield\tIA\tButler County\tH1\n50665\t19023\tParkersburg\tIA\tButler County\tH1\n50611\t19023\tBristow\tIA\tButler County\tH1\n50608\t19023\tAustinville\tIA\tButler County\tH1\n50649\t19023\tKesley\tIA\tButler County\tH1\n50658\t19023\tNashua\tIA\tButler County\tH1\n50604\t19023\tAplington\tIA\tButler County\tH1\n50660\t19023\tNew hartford\tIA\tButler County\tH1\n50579\t19025\tRockwell city\tIA\tCalhoun County\tH1\n50586\t19025\tSomers\tIA\tCalhoun County\tH1\n51433\t19025\tAuburn\tIA\tCalhoun County\tH1\n50561\t19025\tLytton\tIA\tCalhoun County\tH1\n50540\t19025\tFonda\tIA\tCalhoun County\tH1\n51453\t19025\tLohrville\tIA\tCalhoun County\tH1\n50050\t19025\tChurdan\tIA\tCalhoun County\tH1\n50566\t19025\tMoorland\tIA\tCalhoun County\tH1\n51449\t19025\tLake city\tIA\tCalhoun County\tH1\n50563\t19025\tManson\tIA\tCalhoun County\tH1\n50552\t19025\tKnierim\tIA\tCalhoun County\tH1\n50575\t19025\tPomeroy\tIA\tCalhoun County\tH1\n50538\t19025\tFarnhamville\tIA\tCalhoun County\tH1\n50551\t19025\tJolley\tIA\tCalhoun County\tH1\n51466\t19027\tWall lake\tIA\tCarroll County\tH1\n51440\t19027\tDedham\tIA\tCarroll County\tH1\n51452\t19027\tLidderdale\tIA\tCarroll County\tH1\n51453\t19027\tLohrville\tIA\tCarroll County\tH1\n50050\t19027\tChurdan\tIA\tCarroll County\tH1\n51443\t19027\tGlidden\tIA\tCarroll County\tH1\n51430\t19027\tArcadia\tIA\tCarroll County\tH1\n51455\t19027\tManning\tIA\tCarroll County\tH1\n51459\t19027\tRalston\tIA\tCarroll County\tH1\n51401\t19027\tCarroll\tIA\tCarroll 
